vi "Unflatten Value.vi"(8 "Error In":errorcluster, 10 "Value":string, 11 "2D Flt In":refnum<class "2D Flt.lvclass">) -> (0 "Error Out":errorcluster, 3 "2D Flt Out":refnum<class "2D Flt.lvclass">)   [LabVIEW 2020, in "NI_VIAnCFGDataStructure.lvlib" / "2D Flt.lvclass"]
doc: "Dynamic dispatch interface for unflattening Tree Data classes from string."
uses:
  <vilib>/addons/analyzer/VIAnCFGDataStructure/Data Types/2D Flt/2D Flt.lvclass
  <vilib>/addons/analyzer/VIAnCFGDataStructure/Data Types/2D Flt/2D Flt.lvclass/2D Flt.ctl
  <vilib>/addons/analyzer/VIAnCFGDataStructure/Tree Manager/Tree.lvclass
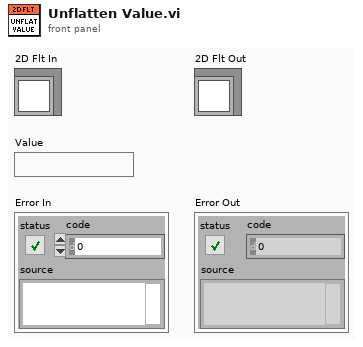
[diagram p1: front panel]
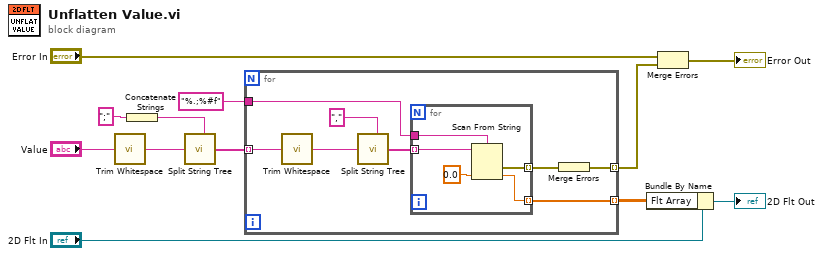
[diagram p0: block diagram]
diagram:
  n1 = call <vilib>:"Trim Whitespace.vi"("string"="Value") -> ("trimmed string"=w1:string)  [unwired: 1 in]
  n2 = Concatenate Strings(";" ("Separator (,)")) -> (w2:string)
  n3 = call <vilib>:"Split String Tree.vi"("Split Pattern"=w2, "Input String"=w1) -> ("Split String"=w12:string[])  [unwired: 5 in]
  n4 = for {
    tunnel: w12 -> [w18] mode=indexing
    tunnel: [w20] -> w11 mode=indexing
    tunnel: [w15] -> w10 mode=indexing
    tunnel: "%.;%#f" ("initial string") -> [w14]
    n5 = call <vilib>:"Trim Whitespace.vi"("string"=w18) -> ("trimmed string"=w13:string)  [unwired: 1 in]
    n6 = call <vilib>:"Split String Tree.vi"("Split Pattern"=",", "Input String"=w13) -> ("Split String"=w17:string[])  [unwired: 5 in]
    n7 = for {
      tunnel: w17 -> [w25] mode=indexing
      tunnel: [w23] -> w20 mode=indexing
      tunnel: [w22] -> w16 mode=indexing
      tunnel: w14 -> [w21]
      n8 = Scan From String(format string=w21, input string=w25, default 1=0.0) -> (error out=w22:errorcluster, output 1=w23:dbl)  [unwired: 2 in, 2 out]
    }
    n9 = Merge Errors(w16) -> (w15:errorcluster)
  }
  n10 = Bundle By Name(cluster="2D Flt In", "Flt Array"=w11) -> (→"2D Flt Out":refnum<class "2D Flt.lvclass">)
  n11 = Merge Errors("Error In", w10) -> (→"Error Out":errorcluster)
